vi "getDeviceType.vi"(8 "error in (no error)":errorcluster, 11 "AoDeviceData in":refnum<class "AoDeviceData.lvclass">) -> (0 "error out":errorcluster, 2 "type":T1(ring), 3 "AoDeviceData out":refnum<class "AoDeviceData.lvclass">)   [LabVIEW 2009, in "DataMappers.lvlib" / "AoDeviceData.lvclass"]
uses:
  AoDeviceData.lvclass
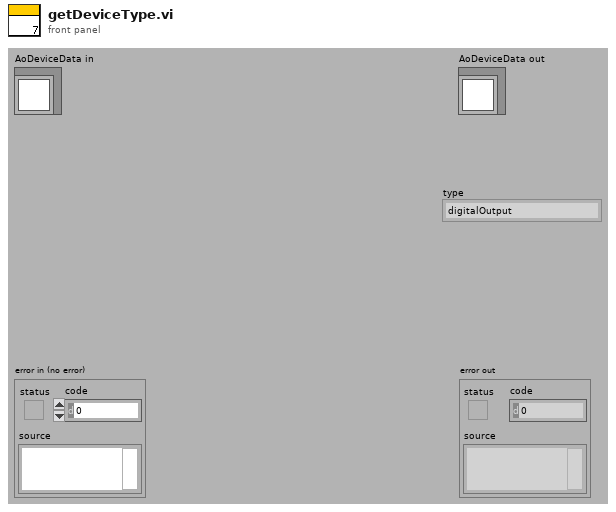
[diagram p1: front panel]
types:
  T1 = enum16{"digitalOutput", "digitalInput", "analogOutput", "analogInput", "rfOutput", "ethernetSupply"}
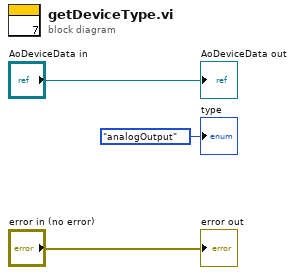
[diagram p0: block diagram]
diagram:
  "error out" <- "error in (no error)"
  "AoDeviceData out" <- "AoDeviceData in"
  "type" <- T1."analogOutput" ("type")
